vi "device_global.vi"() -> ()   [LabVIEW 2019]
uses:
  RHEODYNE7970_ADN.llb/RD7970ADN.lvclass
  MSP1C2.llb/MSP1C2.lvclass
  TETECH_TC720.llb/TC720.lvclass
  SC300.llb/SC300.lvclass
  CAVRO_XC.llb/XC3P.lvclass
  KQZ1-MP.llb/KQZ1.lvclass
  SV_LG16ch.llb/SV_LG16ch.lvclass
  MSST5.llb/MSST5.lvclass
  ST_RMDS.llb/RMDS.lvclass
  PD.llb/PD.lvclass
  VICI EMHCA.llb/VICI EMHCA_10PORTS.lvclass
panel:
  in  "ASI_VISA":refnum<visa-resource-name>
  in  "VICI_EMHCA":refnum<class "VICI EMHCA_10PORTS.lvclass">[](array[class])
  in  "PWD 2":path
  out "TC":bool
  in  "wait":bool
  out "queue scan":refnum<queue>
  in  "PD":refnum<class "PD.lvclass">
  in  "RMDS":refnum<class "RMDS.lvclass">[](array[class])
  in  "Axis_Y":u32
  in  "Axis_X":u32
  in  "lastZ":dbl
  in  "MSST5":refnum<class "MSST5.lvclass">[](array[class])
  in  "SV":refnum<class "SV_LG16ch.lvclass">[](array[class])
  in  "KQZ1.lvclass":refnum<class "KQZ1.lvclass">
  in  "PP_KQZ1":refnum<class "KQZ1.lvclass">[](array[class])
  in  "XC3P.lvclass":refnum<class "XC3P.lvclass">
  in  "SP_XC":refnum<class "XC3P.lvclass">[](array[class])
  in  "PWD":path
  in  "ST_SC300":refnum<class "SC300.lvclass">[](array[class])
  out "Boolean":bool
  in  "TC_TC720":refnum<class "TC720.lvclass">[](array[class])
  in  "RV_RD7970ADN":refnum<class "RD7970ADN.lvclass">[](array[class])
  in  "SP_MSP1C2":refnum<class "MSP1C2.lvclass">[](array[class])
  in  "SP1":refnum<class "MSP1C2.lvclass">
  in  "RV1":refnum<class "RD7970ADN.lvclass">
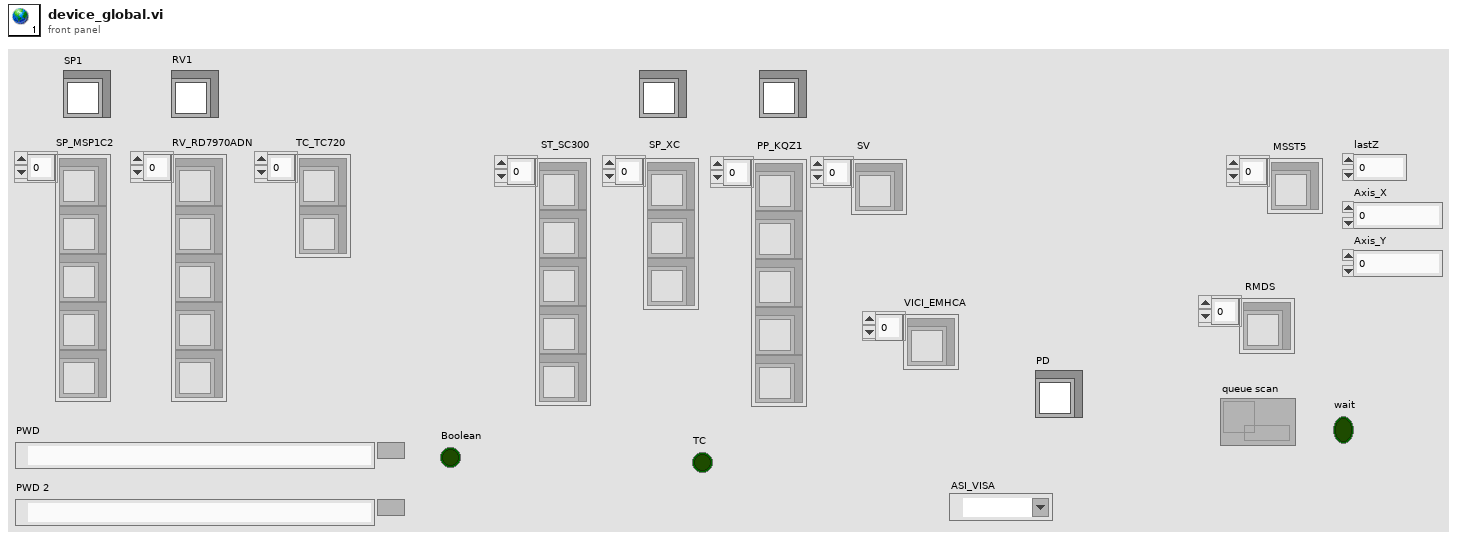
[diagram p1: front panel]
diagram:
